vi "Create RawPhase, TTL, Extracted Phase from Raw Phase Data.vi"(0 "sampling info":cluster{"Fs":dbl, "#s":dbl}={"Fs"=100000000.0, "#s"=1000000.0}, 5 "sampling freq: fs":dbl=80000.0, 7 "Raw Input Data":dbl[][](array[numeric]), 9 "order":i32=2, 11 "dt":dbl=1e-08, 12 "low cutoff freq: fl":dbl=10.0) -> (3 "Squeezing Arches Phase":dbl[](graph), 4 "detected frequency":dbl format="%.4p", 6 "detected phase (deg)":dbl format="%.2p", 8 "Output Data":dbl[][](array[numeric]), 10 "Envelope":dbl[](graph), 14 "Phase Array of Squeezed Pulses":dbl[](array[numeric]), 15 "Normalized Envelope":waveform(dbl)(graph))   [LabVIEW 2009]
panel:
  # "Raw Arches"
  # "TTL"
  # "Phase"
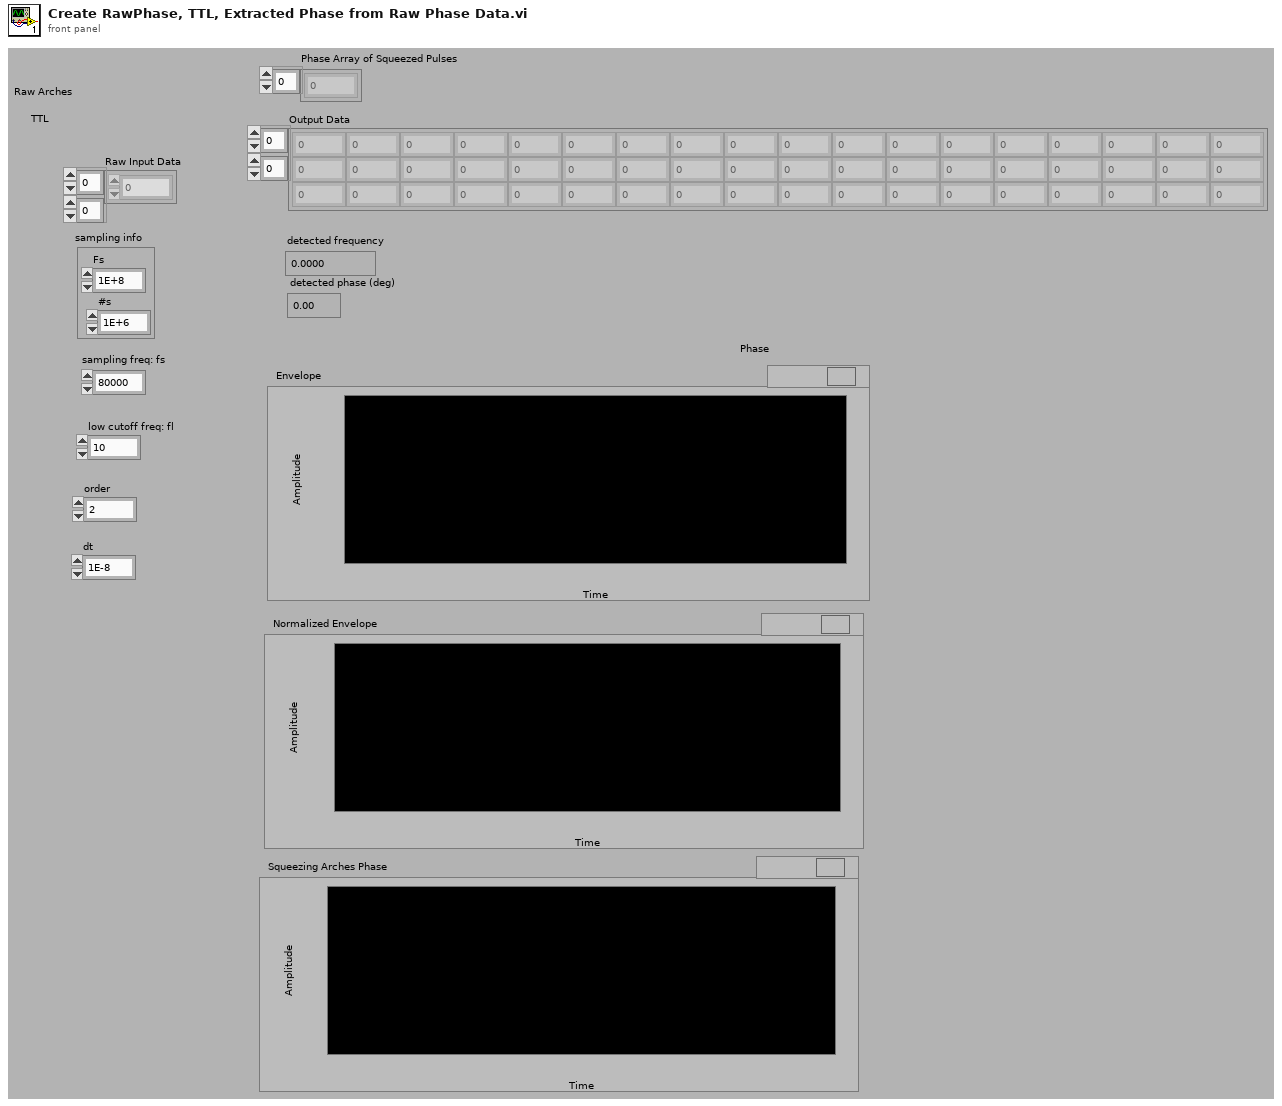
[diagram p1: front panel]
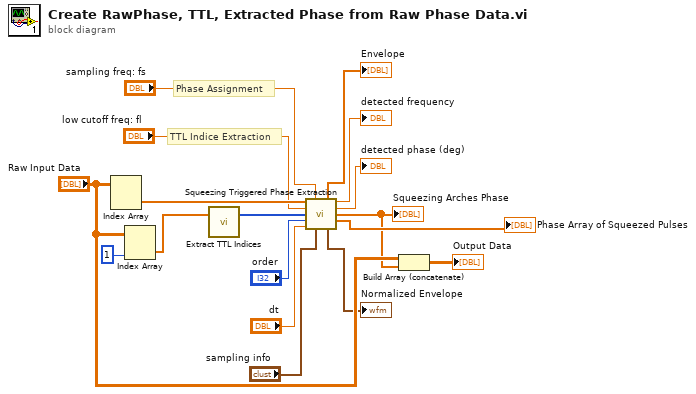
[diagram p0: block diagram]
diagram:
  # "TTL Indice Extraction"
  # "Phase Assignment"
  n1 = Index Array(array="Raw Input Data") -> (element=w12:dbl[])  [unwired: 2 in]
  n2 = Index Array(array="Raw Input Data", index (col)=1 ("disabled index (col)")) -> (element=w13:dbl[])  [unwired: 1 in]
  n3 = call "Extract TTL Indices.vi"("Analog TTL"=w13) -> ("Rising Transition Indices"=w14:u32[])  [unwired: 1 in, 1 out]
  n4 = call "Squeezing Triggered Phase Extraction.vi"("Input Data"=w12, "sampling freq: fs"="sampling freq: fs", "low cutoff freq: fl"="low cutoff freq: fl", "Measurement indices"=w14, "order"="order", "dt"="dt", "sampling info"="sampling info") -> ("Envelope"=→"Envelope":dbl[], "detected frequency"=→"detected frequency":dbl, "detected phase (deg)"=→"detected phase (deg)":dbl, "Squeezing Arches Phase Array"=w1:dbl[], "Phase Array of Squeezed Pulses"=→"Phase Array of Squeezed Pulses":dbl[], "Normalized Envelope"=→"Normalized Envelope":waveform(dbl))  [unwired: 3 in]
  "Squeezing Arches Phase" <- w1
  n5 = Build Array (concatenate)("Raw Input Data", w1) -> (→"Output Data":dbl[][])
